vi "_Test Executor.vi"() -> ()   [LabVIEW 2021]
uses:
  Typedef/Def-Executor Command.ctl
  Typedef/Def-LogSpec.ctl
  Typedef/Def-CAN Port Configuration.ctl
  XNET-CAN-Signal-Logger.lvlib
panel:
  out "error out":errorcluster
  in  "test user event":bool
  in  "destroy user event":bool
  out "current time":timestamp
  in  "exit":bool
  in  "stop logging":bool
  in  "start logging":bool
  in  "config":bool
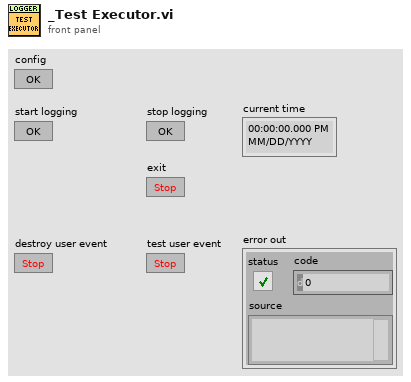
[diagram p1: front panel]
types:
  T1 = typedef "XNET-CAN-Signal-Logger.lvlib/Def-LogSpec.ctl" = cluster{"Log file folder":path, "Log file name":string, "Segment Files":bool, "Segment File Size":i64}
  T2 = typedef "XNET-CAN-Signal-Logger.lvlib/Def-CAN Port Configuration.ctl" = cluster{"CAN Interface":refnum<k21>, "XNET Cluster":refnum<k21>, "#Signals":i32, "Sample Rate (Hz)":dbl}
  T3 = cluster{"LogSpec":T1, "CAN Configurations out":T2[]}
  T4 = typedef "XNET-CAN-Signal-Logger.lvlib/Def-Executor Command.ctl" = cluster{"Command":string, "Data":variant}
  T5 = cluster{"LogSpec out":T1, "CAN Configurations out":T2[]}
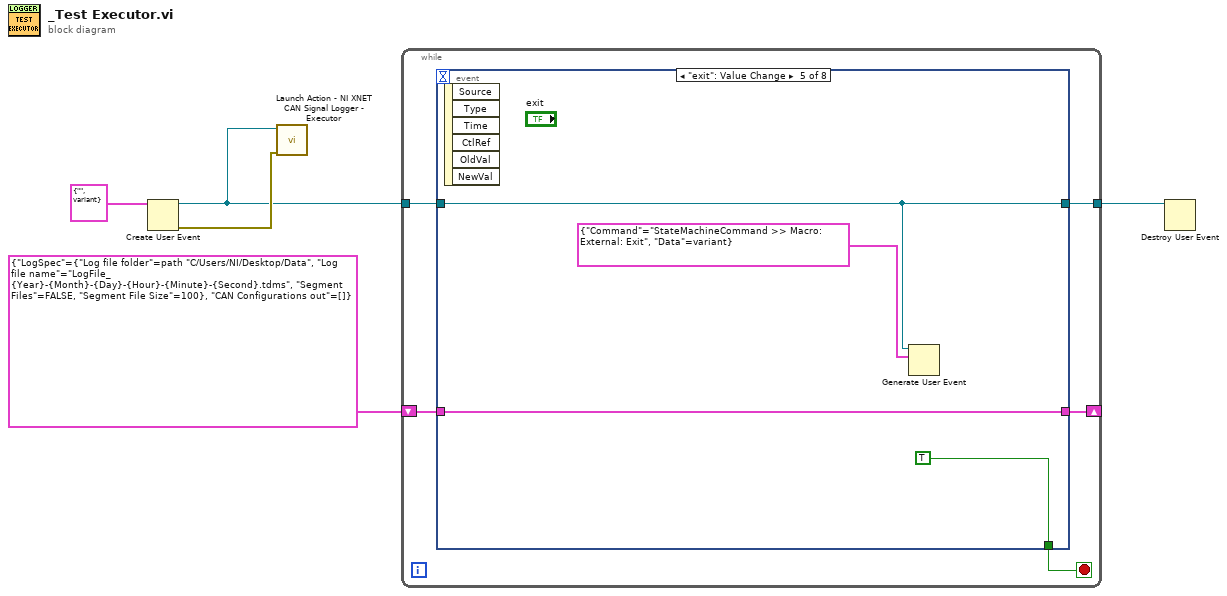
[diagram p0: block diagram]
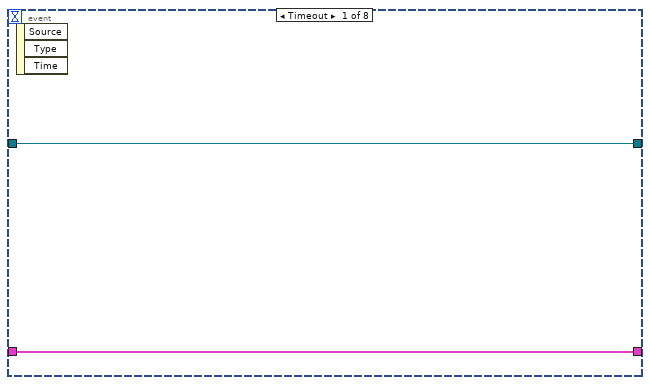
[diagram p2: hidden frame]
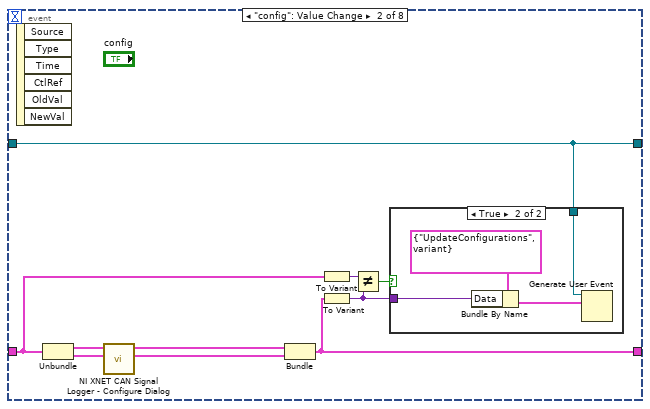
[diagram p3: hidden frame]
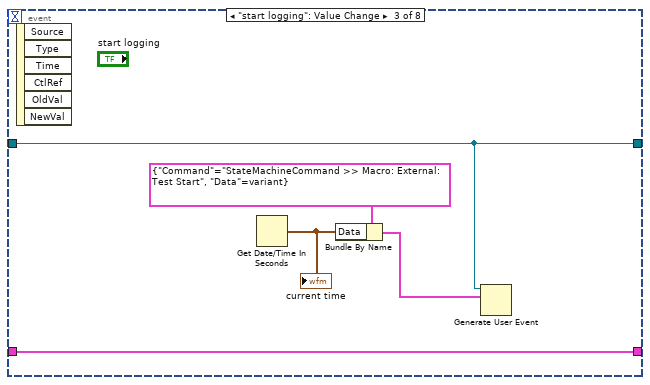
[diagram p5: hidden frame]
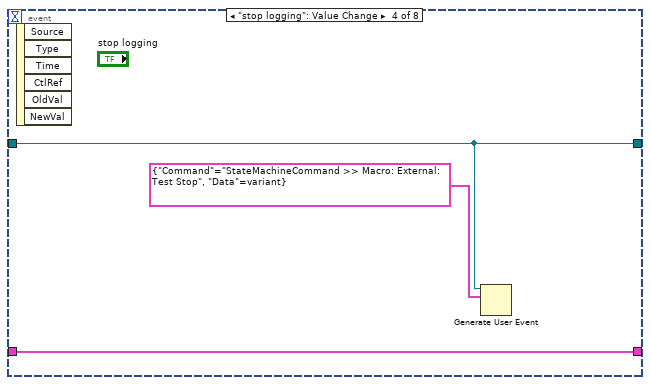
[diagram p6: hidden frame]
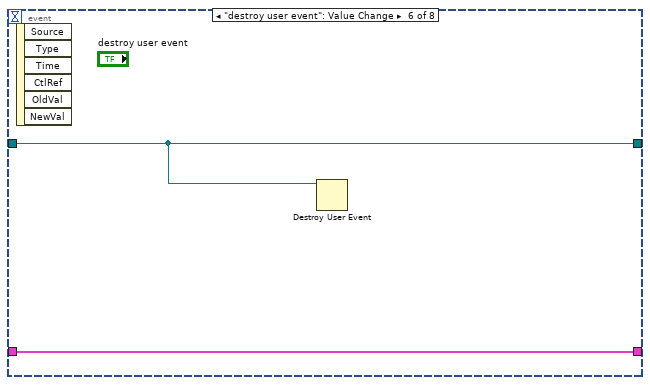
[diagram p7: hidden frame]
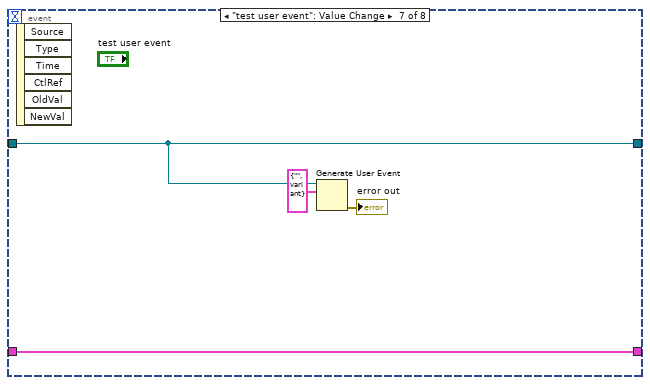
[diagram p8: hidden frame]
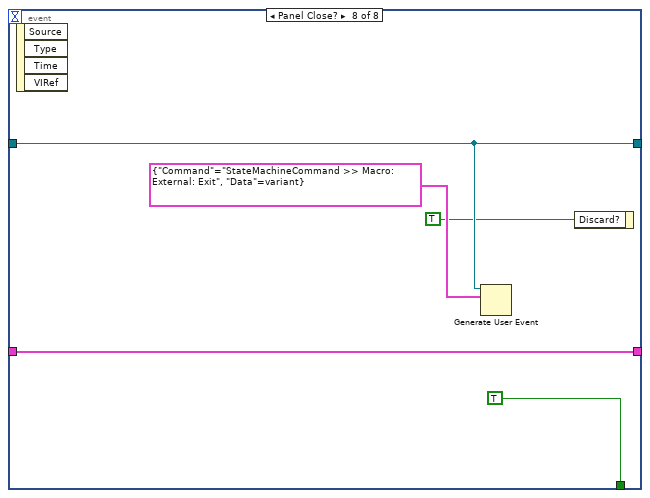
[diagram p9: hidden frame]
diagram:
  n1 = Create User Event(user event datatype=T4 {"Command"="", "Data"=variant} ("Command")) -> (user event=w3:refnum<user-event>, error out=w4:errorcluster)  [unwired: 1 in]
  n2 = call "Launch Action - NI XNET CAN Signal Logger - Executor.vi"("error in (no error)"=w4, "Executor Command"=w3) -> ()  [unwired: 9 in, 1 out]
  n3 = while {
    tunnel: w3 -> [w10]
    tunnel: [w8] -> w2
    shift-right: [w7] -> _
    shift-left: T3 {"LogSpec"={"Log file folder"=path "C:/Users/NI/Desktop/Data", "Log file name"="LogFile_{Year}-{Month}-{Day}-{Hour}-{Minute}-{Second}.tdms", "Segment Files"=FALSE, "Segment File Size"=100}, "CAN Configurations out"=[]} -> [w6]
    stop <- w9 stop-if-true
    n4 = event shown="[4] \"exit\": Value Change" {
      selector: _ -> [_ _ _ _ _ _ _ _]
      dyn-events: _ -> [_ _ _ _ _ _ _ _]
      timeout: _ -> [_ _ _ _ _ _ _ _]
      tunnel: w10 -> [w12 w22 w29 w33 w37 w39 w43 w48]
      tunnel: [_ _ _ _ TRUE _ _ TRUE] -> w9
      tunnel: [w12 w22 w29 w33 w37 w39 w43 w48] -> w8
      tunnel: [w11 w20 w28 w32 w35 w40 w44 w45] -> w7
      tunnel: w6 -> [w11 w17 w28 w32 w35 w40 w44 w45]
      event Timeout {
        n5 = event-data() -> ()  [unwired: 1 in, 3 out]
      }
      event "config": Value Change {
        n6 = event-data() -> ()  [unwired: 1 in, 6 out]
        n7 = Unbundle(w17) -> ("LogSpec"=w19:T1, "CAN Configurations out"=w18:T2[])
        n8 = call "NI XNET CAN Signal Logger - Configure Dialog.vi"("CAN Configurations in"=w18, "LogSpec in"=w19) -> ("CAN Configurations out"=w13:T2[], "LogSpec out"=w21:T1)  [unwired: 7 in, 1 out]
        n9 = Bundle("LogSpec out"=w21, "CAN Configurations out"=w13) -> (w20:T5)  [unwired: 1 in]
        n10 = To Variant(anything=w17) -> (Variant=w16:variant)
        n11 = To Variant(anything=w20) -> (Variant=w15:variant)
        n12 = Not Equal?(x=w16, y=w15) -> (x != y?=w14:bool)
        n13 = case shown="True" w14 {
          tunnel: w22 -> [_ w24]
          tunnel: w15 -> [_ w23]
          frame False {
          }
          frame True {
            n14 = Bundle By Name(cluster=T4 {"Command"="UpdateConfigurations", "Data"=variant} ("event data"), "Data"=w23) -> (w25:T4)
            n15 = Generate User Event(user event=w24, event data cluster=w25) -> ()  [unwired: 2 in, 2 out]
          }
        }
      }
      event "start logging": Value Change {
        n16 = event-data() -> ()  [unwired: 1 in, 6 out]
        n17 = Get Date/Time In Seconds() -> (seconds since 1Jan1904=w27:timestamp)
        "current time" <- w27
        n18 = Bundle By Name(cluster=T4 {"Command"="StateMachineCommand >> Macro: External: Test Start", "Data"=variant} ("event data"), "Data"=w27) -> (w30:T4)
        n19 = Generate User Event(user event=w29, event data cluster=w30) -> ()  [unwired: 2 in, 2 out]
      }
      event "stop logging": Value Change {
        n20 = event-data() -> ()  [unwired: 1 in, 6 out]
        n21 = Generate User Event(user event=w33, event data cluster=T4 {"Command"="StateMachineCommand >> Macro: External: Test Stop", "Data"=variant} ("event data")) -> ()  [unwired: 2 in, 2 out]
      }
      event "exit": Value Change {
        n22 = event-data() -> ()  [unwired: 1 in, 6 out]
        n23 = Generate User Event(user event=w37, event data cluster=T4 {"Command"="StateMachineCommand >> Macro: External: Exit", "Data"=variant} ("event data")) -> ()  [unwired: 2 in, 2 out]
      }
      event "destroy user event": Value Change {
        n24 = event-data() -> ()  [unwired: 1 in, 6 out]
        n25 = Destroy User Event(user event=w39) -> ()  [unwired: 1 in, 1 out]
      }
      event "test user event": Value Change {
        n26 = event-data() -> ()  [unwired: 1 in, 6 out]
        n27 = Generate User Event(user event=w43, event data cluster=T4 {"Command"="", "Data"=variant} ("event data")) -> (error out=→"error out":errorcluster)  [unwired: 2 in, 1 out]
      }
      event Panel Close? {
        n28 = event-data() -> ()  [unwired: 1 in, 4 out]
        n29 = Generate User Event(user event=w48, event data cluster=T4 {"Command"="StateMachineCommand >> Macro: External: Exit", "Data"=variant} ("event data")) -> ()  [unwired: 2 in, 2 out]
        n30 = event-data("Discard?"=TRUE) -> ()  [unwired: 1 in, 1 out]
      }
    }
  }
  n31 = Destroy User Event(user event=w2) -> ()  [unwired: 1 in, 1 out]
